vi "properties.from_json.vi"(8 "error in":errorcluster, 10 "json":string) -> (0 "error out":errorcluster, 2 "properties":T1)   [LabVIEW 2020, in "type.lvclass"]
uses:
  property.ctl
  property value.ctl
  <vilib>/JDP Science/JSONtext/Variant to JSON Text.vi
  <vilib>/JDP Science/JSONtext/LVClass Serializer/JSONtext LVClass Serializer.lvclass
  type.lvclass
  type.lvclass/type.ctl
  <vilib>/JDP Science/JSONtext/JSONtext.lvlib
  1faf4446-3ada-4580-8778-cf8f364cebb8.vi
  properties.ctl
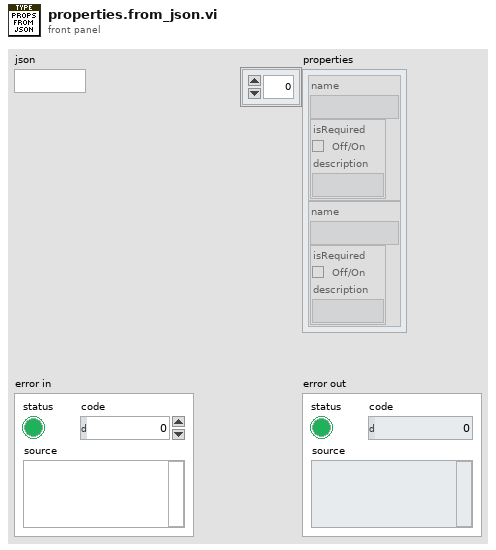
[diagram p1: front panel]
types:
  T1 = typedef "type.lvclass/properties.ctl" = T2[]
  T2 = typedef "type.lvclass/property.ctl" = cluster{"name":string, "value":T3}
  T3 = typedef "type.lvclass/property value.ctl" = cluster{"isRequired":bool, "description":string}
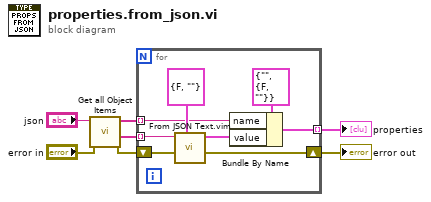
[diagram p0: block diagram]
diagram:
  n1 = call <vilib>:"Get all Object Items.vi"("error in (no error)"="error in", "JSON"="json") -> ("error out"=w3:errorcluster, "<JSON>"=w5:string[], "Item Names"=w6:string[])  [unwired: 6 in, 1 out]
  n2 = for {
    tunnel: w6 -> [w13] mode=indexing
    tunnel: w5 -> [w14] mode=indexing
    tunnel: [w10] -> w4 mode=indexing
    shift-right: [w9] -> w1
    shift-left: w3 -> [w8]
    n3 = call "From JSON Text.vim"("Data Type and Default Value"=T3 {"isRequired"=FALSE, "description"=""} ("value"), "error in (no error)"=w8, "JSON"=w14) -> ("error out"=w9:errorcluster, "Data out"=w12:T3)  [unwired: 7 in]
    n4 = Bundle By Name(cluster=T2 {"name"="", "value"={"isRequired"=FALSE, "description"=""}} ("Cluster"), "name"=w13, "value"=w12) -> (w10:T2)
  }
  "properties" <- w4
  "error out" <- w1
